vi "Analyze.vi"(8 "error in (no error)":errorcluster, 10 "Image in":T1, 11 "Analyze Fluence and Energy in":refnum<class "Analyze Fluence and Energy.lvclass">) -> (0 "error out":errorcluster, 1 "Result":refnum<class "Analyze Results Base.lvclass">, 2 "Image out":T1, 3 "Analyze Fluence and Energy out":refnum<class "Analyze Fluence and Energy.lvclass">)   [LabVIEW 2020, in "Analyze.lvlib" / "Analyze Fluence and Energy.lvclass"]
uses:
  Analyze Fluence and Energy.lvclass
  C:/POLARIS Programme/POLARIS-AS-3-Cams/Submodules/HIJ Vision/Analyze/Analyze Classes/Analyze BaseClass/Analyze BaseClass/Analyze BaseClass.lvclass
  <vilib>/vision/Image Controls.llb/IMAQ Image.ctl
  Results and Overlays/Results Base/Analyze Results Base.lvclass
  Analyze Energy/Analyze Energy.lvclass
  Analyze Fluence/Analyze Fluence.lvclass
  Results and Overlays/Results Fluence and Energy/Analyze Results Fluence and Energy.lvclass
  C:/POLARIS Programme/POLARIS-AS-3-Cams/Submodules/HIJ Vision/Analyze/Results and Overlays/Results Base/Analyze Results Base.lvclass
  C:/POLARIS Programme/POLARIS-AS-3-Cams/Submodules/HIJ Vision/Analyze/Results and Overlays/Compound Results/Analyze Compound Results Base.lvclass
  Results and Overlays/Results Energy/Analyze Results Energy.lvclass/Analyze Results Energy.ctl
  Results and Overlays/Results Energy/Read Energy.vi
  Results and Overlays/Results Fluence/Analyze Results Fluence.lvclass
  Results and Overlays/Results Energy/Analyze Results Energy.lvclass
  Analyze Compound Analysis Base/Analyze Compound Analysis Base.lvclass
  Analyze BaseClass/Analyze BaseClass/Analyze BaseClass.lvclass
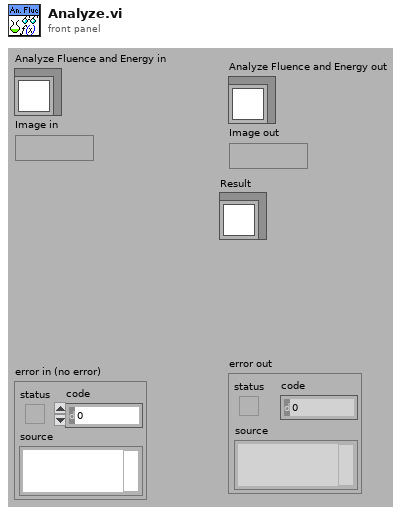
[diagram p1: front panel]
types:
  T1 = typedef "IMAQ Image.ctl" = refnum<image>
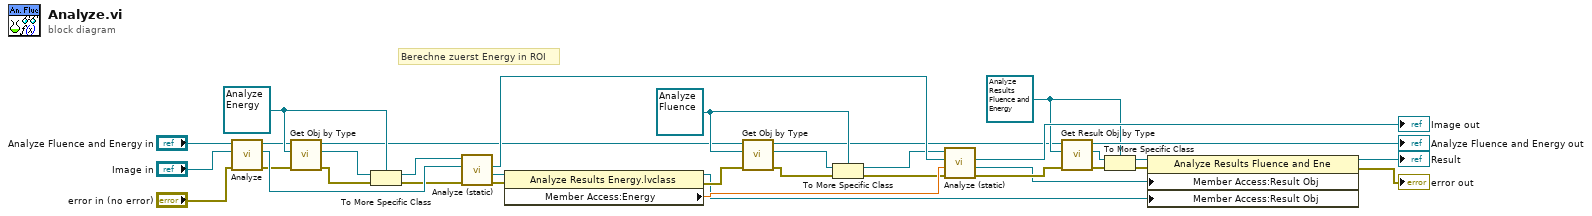
[diagram p0: block diagram]
diagram:
  w25 = refnum<class "Analyze Results Fluence and Energy.lvclass"> refnum ("Analyze Results Fluence and Energy.lvclass")
  w35 = refnum<class "Analyze Fluence.lvclass"> refnum ("Analyze.lvlib:Analyze Fluence.lvclass")
  w30 = refnum<class "Analyze Energy.lvclass"> refnum ("Analyze.lvlib:Analyze Energy.lvclass")
  # "Berechne zuerst Energy in ROI"
  n1 = call-parent "Analyze.vi"("error in (no error)"="error in (no error)", "Image in"="Image in", "Analyze BaseClass in"="Analyze Fluence and Energy in") -> ("error out"=w6:errorcluster, "Image out"=w20:T1, "Analyze BaseClass out"=w17:refnum<class "Analyze Fluence and Energy.lvclass">)  [unwired: 5 in, 1 out]
  n2 = call-dynamic "Get Obj by Type.vi"("error in (no error)"=w6, "Type"=w30, "Analyze Compound Analysis Base in"=w17) -> ("error out"=w5:errorcluster, "Analyze Obj"=w16:refnum<class "Analyze BaseClass.lvclass">, "Analyze Compound Analysis Base out"=w12:refnum<class "Analyze Fluence and Energy.lvclass">)  [unwired: 5 in, 1 out]
  n3 = To More Specific Class(target class=w30, reference=w16, error in=w5) -> (specific class reference=w14:refnum<class "Analyze Energy.lvclass">, error out=w15:errorcluster)
  n4 = call "Analyze (static).vi"("error in (no error)"=w15, "Image in"=w20, "Analyze Energy in"=w14) -> ("error out"=w19:errorcluster, "Result"=w18:refnum<class "Analyze Results Energy.lvclass">, "Image out"=w21:T1)  [unwired: 5 in, 1 out]
  n5 = property class="Analyze Results Energy.lvclass"(reference=w18, error in=w19) -> (reference out=w2:refnum<class "Analyze Results Energy.lvclass">, error out=w8:errorcluster, "Member Access:Energy"=w10:dbl[unit])
  n6 = call-dynamic "Get Obj by Type.vi"("error in (no error)"=w8, "Type"=w35, "Analyze Compound Analysis Base in"=w12) -> ("error out"=w9:errorcluster, "Analyze Obj"=w13:refnum<class "Analyze BaseClass.lvclass">, "Analyze Compound Analysis Base out"=w4:refnum<class "Analyze Fluence and Energy.lvclass">)  [unwired: 5 in, 1 out]
  n7 = To More Specific Class(target class=w35, reference=w13, error in=w9) -> (specific class reference=w11:refnum<class "Analyze Fluence.lvclass">, error out=w7:errorcluster)
  n8 = call "Analyze (static).vi"("error in (no error)"=w7, "Energy"=w10, "Image in"=w21, "Analyze Fluence in"=w11) -> ("error out"=w3:errorcluster, "Result"=w1:refnum<class "Analyze Results Fluence.lvclass">, "Image out"=→"Image out":T1)  [unwired: 4 in, 1 out]
  n9 = call "Get Result Obj by Type.vi"("error in (no error)"=w3, "Parameter Type"=w25, "Analyze BaseClass in"=w4) -> ("error out"=w24:errorcluster, "Parameter"=w28:refnum<class "Analyze Results Base.lvclass">, "Analyze BaseClass out"=→"Analyze Fluence and Energy out":refnum<class "Analyze Fluence and Energy.lvclass">)  [unwired: 5 in, 1 out]
  n10 = To More Specific Class(target class=w25, reference=w28, error in=w24) -> (specific class reference=w26:refnum<class "Analyze Results Fluence and Energy.lvclass">, error out=w23:errorcluster)
  n11 = property class="Analyze Results Fluence and Ene"(reference=w26, error in=w23, "Member Access:Result Obj"=w1, "Member Access:Result Obj"=w2) -> (reference out=→"Result":refnum<class "Analyze Results Fluence and Energy.lvclass">, error out=→"error out":errorcluster)
